vi "Map.vi"(7 "Action":enum8{"noop", "get", "set", "pop"}(ring), 10 "App in":T1, 11 "App ID in":u16) -> (1 "Found?":bool, 2 "App out":T1, 3 "App ID out":u16)   [LabVIEW 2018, in "TCPServer.lvlib"]
uses:
  TCPServer.lvlib
  TypeDefs/Connection.ctl
  TypeDefs/App.ctl
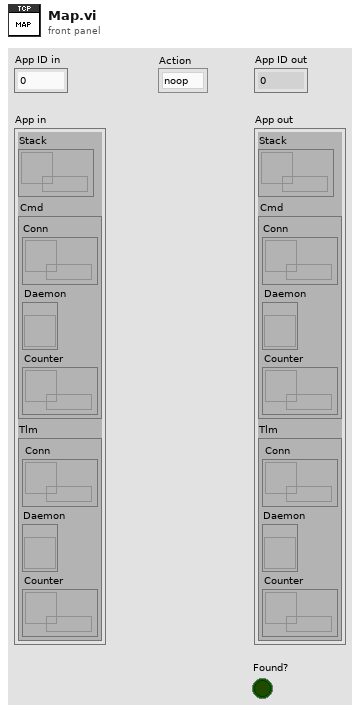
[diagram p1: front panel]
types:
  T1 = typedef "TCPServer.lvlib/App.ctl" = cluster{"Stack":refnum<queue>, "Cmd":cluster{"Conn":refnum<data-value>, "Daemon":refnum<vi>, "Counter":refnum<data-value>}, "Tlm":cluster{"Conn":refnum<data-value>, "Daemon":refnum<vi>, "Counter":refnum<data-value>}}
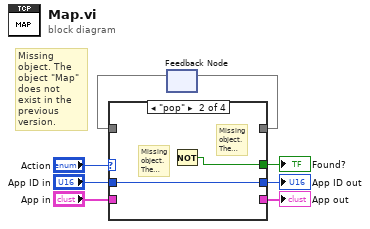
[diagram p0: block diagram]
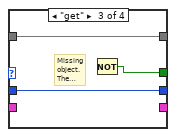
[diagram p3: hidden frame]
diagram:
  # "Missing object. The object \"Map\" does not exist in the previous version."
  n1 = feedback #1() -> (w6, w5)
  n2 = case shown="\"pop\"" "Action" {
    tunnel: [w12 _ w22 w26] -> w7
    tunnel: "App in" -> [w10 w15 w21 w24]
    tunnel: w6 -> [w12 w17 w22 w27]
    tunnel: "App ID in" -> [w11 w16 w19 w25]
    tunnel: [w11 w16 w19 w25] -> w3
    tunnel: [w10 w14 w20 w24] -> w2
    tunnel: [_ w13 w18 w23] -> w1
    frame "noop" {
    }
    frame "pop" {
      # "Missing object. The object \"Remove From Map\" does not exist in the previous version."
      # "Missing object. The object \"Look In Map\" does not exist in the previous version."
      n3 = Not() -> (.not. x?=w13:bool)  [unwired: 1 in]
    }
    frame "get" {
      # "Missing object. The object \"Look In Map\" does not exist in the previous version."
      n4 = Not() -> (.not. x?=w18:bool)  [unwired: 1 in]
    }
    frame "set" {
      # "Missing object. The object \"Insert Into Map\" does not exist in the previous version."
    }
  }
  "App out" <- w2
  "App ID out" <- w3
  "Found?" <- w1
  n5 = feedback-in #1(w7) -> ()
